vi "Device data to Plot.vi"(8 "Error In":errorcluster, 9 "Device Data array":T1[](array[typedef]) {"Data" format="%#_6f"}, 10 "Hum Plot Reference":refnum<vi>, 11 "Temp Plot Reference":refnum<vi>) -> (0 "Error Out":errorcluster, 1 "Hum Plot":cluster{"Array":dbl[], "Array":dbl[]}[](array[cluster]), 2 "Temp Plot":cluster{"Array":dbl[], "Array":dbl[]}[](array[cluster]))   [LabVIEW 2016]
uses:
  Typedef/Device data.ctl
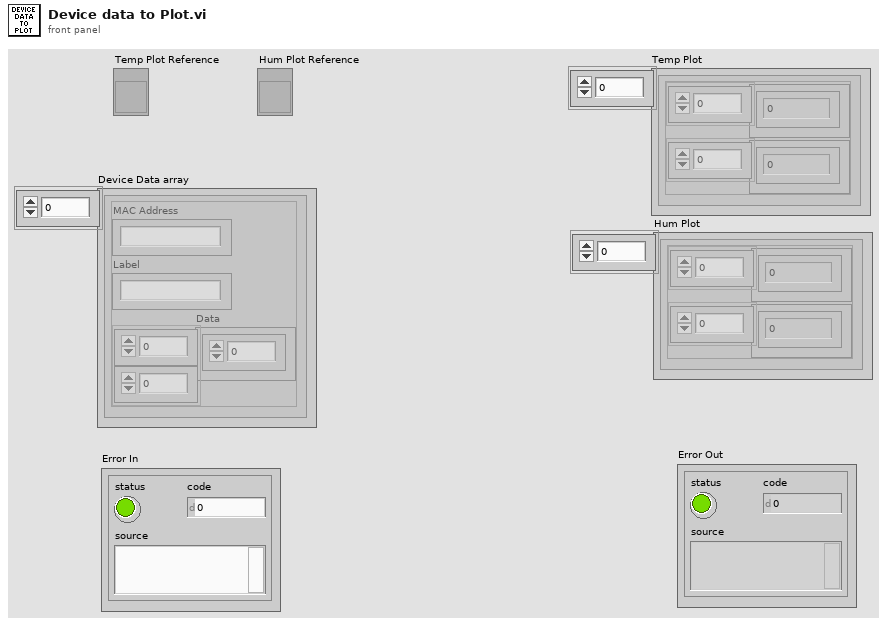
[diagram p1: front panel]
types:
  T1 = typedef "Device data.ctl" = cluster{"MAC Address":string, "Label":string, "Data":dbl[][]}
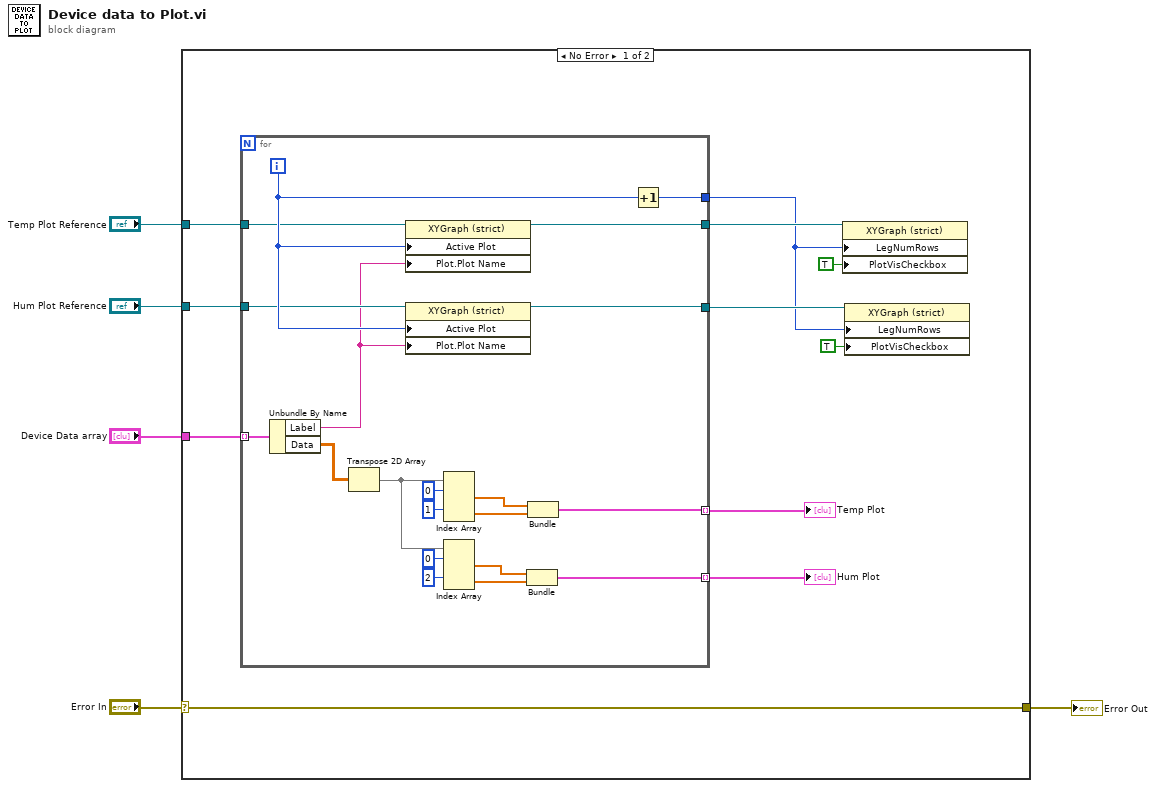
[diagram p0: block diagram]
diagram:
  n1 = case shown="No Error" "Error In" {
    selector: "Error In" -> [w16 w37]
    tunnel: [w16 w37] -> w4
    tunnel: "Device Data array" -> [w15 _]
    tunnel: "Temp Plot Reference" -> [w14 _]
    tunnel: "Hum Plot Reference" -> [w13 _]
    frame No Error {
      n2 = for {
        tunnel: w15 -> [w36] mode=indexing
        tunnel: [w23] -> w10
        tunnel: [w25] -> w7 mode=indexing
        tunnel: [w24] -> w6 mode=indexing
        tunnel: w14 -> [w21]
        tunnel: w13 -> [w20]
        tunnel: [w18] -> w12
        tunnel: [w17] -> w11
        i -> [w22]
        n3 = Unbundle By Name(w36) -> ("Label"=w19:string, "Data"=w35:dbl[][])
        n4 = Transpose 2D Array(2D array=w35) -> (transposed array=w30:dbl[][])
        n5 = property class="XYGraph (strict)"(reference=w21, "Active Plot"=w22, "Plot.Plot Name"=w19) -> (reference out=w18:refnum<vi>)  [unwired: 1 in, 1 out]
        n6 = property class="XYGraph (strict)"(reference=w20, "Active Plot"=w22, "Plot.Plot Name"=w19) -> (reference out=w17:refnum<vi>)  [unwired: 1 in, 1 out]
        n7 = Index Array(array=w30, index (row) #1=0 ("index (row)"), index (row) #2=1 ("index (row)")) -> (element #1=w29:dbl[], element #2=w28:dbl[])  [unwired: 2 in]
        n8 = Index Array(array=w30, index (row) #1=0 ("index (row)"), index (row) #2=2 ("index (row)")) -> (element #1=w26:dbl[], element #2=w27:dbl[])  [unwired: 2 in]
        n9 = Bundle(w26, w27) -> (w24:cluster{dbl[], dbl[]})  [unwired: 1 in]
        n10 = Bundle(w29, w28) -> (w25:cluster{dbl[], dbl[]})  [unwired: 1 in]
        n11 = Increment(x=w22) -> (x+1=w23:i32)
      }
      "Temp Plot" <- w7
      "Hum Plot" <- w6
      n12 = property class="XYGraph (strict)"(reference=w12, "LegNumRows"=w10, "PlotVisCheckbox"=TRUE ("Legend:Plot Visibility Checkbox Visible")) -> ()  [unwired: 1 in, 2 out]
      n13 = property class="XYGraph (strict)"(reference=w11, "LegNumRows"=w10, "PlotVisCheckbox"=TRUE ("Legend:Plot Visibility Checkbox Visible")) -> ()  [unwired: 1 in, 2 out]
    }
    frame Error {
    }
  }
  "Error Out" <- w4
